vi "S4GUI.vi"(7 "Tab ObsEng":enum32{"Obs", "CCD modes", "Eng"}(tab)) -> ()   [LabVIEW 2018] (continued)
            n1389 = call-dynamic "Read InfoCCDmode.vi"("error in (no error)"=w2404, "S4GUI in"=w2402) -> ("error out"=w2386:errorcluster, "InfoCCDmode"=w2403:T2, "S4GUI out"=w2387:refnum<class "S4GUI.lvclass">)  [unwired: 7 in]
            n1390 = local write "InfoCCDmode"(w2403) -> ()
            n1391 = call-dynamic "CalcTemp.vi"("error in (no error)"=w2386, "S4GUI in"=w2387) -> ("error out"=w2385:errorcluster, "S4GUI out"=w2383:refnum<class "S4GUI.lvclass">)  [unwired: 8 in]
            n1392 = call-dynamic "Read Prev Temp.vi"("error in (no error)"=w2385, "S4GUI in"=w2383) -> ("error out"=w2384:errorcluster, "Prev Temp"=w2381:dbl, "S4GUI out"=w2382:refnum<class "S4GUI.lvclass">)  [unwired: 7 in]
            n1393 = local write "Preview Temp."(w2381) -> ()
          }
          frame "Eng" {
            w2530 = T12."Disabled and Grayed Out" ("Disabled")
            # "Desabilita os botões SET."
            # "Entrou na aba  \"Eng\", ajusta para modo usuário normal..."
            n1394 = local write "password"("" ("password")) -> ()
            n1395 = call-dynamic "Write mode Adm.vi"("error in (no error)"=w2532, "mode Adm"=FALSE, "S4GUI in"=w2533) -> ("error out"=w2525:errorcluster, "S4GUI out"=w2528:refnum<class "S4GUI.lvclass">)  [unwired: 7 in]
            n1396 = property on="Set from Input ch1" class="Bool"("DisabledEnum"=w2530) -> ()  [unwired: 2 in, 2 out]
            n1397 = property on="Set from Input ch3" class="Bool"("DisabledEnum"=w2530) -> ()  [unwired: 2 in, 2 out]
            n1398 = property on="Set from Input ch2" class="Bool"("DisabledEnum"=w2530) -> ()  [unwired: 2 in, 2 out]
            n1399 = property on="Set from Input ch4" class="Bool"("DisabledEnum"=w2530) -> ()  [unwired: 2 in, 2 out]
            n1400 = local read "TARGET NAME WPSEL"() -> (w2481:enum16{"NONE", "OFF", "L/2", "L/4"})
            n1401 = call "Read Instrument.lvclass.vi"("error in (no error)"=w2525, "S4ACS_GUI in"=w2528) -> ("error out"=w2506:errorcluster, "Instrument.lvclass"=w2523:refnum<class "Instrument.lvclass">, "S4ACS_GUI out"=w2527:refnum<class "S4GUI.lvclass">)  [unwired: 7 in]
            n1402 = local read "TARGET NAME CALW"() -> (w2471:T9)
            n1403 = property on="TARGET NAME WPSEL" class="Enum (strict)"() -> ("RingText.Text"=w2479:string)  [unwired: 2 in, 2 out]
            n1404 = call "Read WPSEL.vi"("error in (no error)"=w2506, "Instrument in"=w2523) -> ("error out"=w2521:errorcluster, "Opt_Selector.lvclass"=w2519:refnum<class "Opt_Selector.lvclass">, "Instrument out"=w2522:refnum<class "Instrument.lvclass">)  [unwired: 7 in]
            n1405 = Build Array(-1.0 ("element"), 80.0 ("element"), 0.0 ("element"), 160.0 ("element")) -> (w2482:dbl[])
            n1406 = property on="TARGET NAME CALW" class="Enum (strict)"() -> ("RingText.Text"=w2470:string)  [unwired: 2 in, 2 out]
            n1407 = Build Array(-1.0 ("element"), 0.0 ("element"), 72.0 ("element"), 144.0 ("element"), 216.0 ("element"), 288.0 ("element")) -> (w2474:dbl[])
            n1408 = Index Array "Index Array"(array=w2482, index=w2481) -> (element=w2480:dbl)
            n1409 = call "Write target name.vi"("error in (no error)"=w2521, "target name"=w2479, "Optics in"=w2519) -> ("error out"=w2520:errorcluster, "Optics out"=w2518:refnum<class "Opt_Selector.lvclass">)  [unwired: 7 in]
            n1410 = Index Array(array=w2474, index=w2471) -> (element=w2469:dbl)
            n1411 = call "Write target.vi"("error in (no error)"=w2520, "target"=w2480, "Optics in"=w2518) -> ("error out"=w2516:errorcluster, "Optics out"=w2517:refnum<class "Opt_Selector.lvclass">)  [unwired: 7 in]
            n1412 = call "Write WPSEL.vi"("error in (no error)"=w2516, "Opt_Selector.lvclass"=w2517, "Instrument in"=w2522) -> ("error out"=w2515:errorcluster, "Instrument out"=w2514:refnum<class "Instrument.lvclass">)  [unwired: 7 in]
            n1413 = call "Read CALW.vi"("error in (no error)"=w2515, "Instrument in"=w2514) -> ("error out"=w2512:errorcluster, "Opt_Selector.lvclass"=w2510:refnum<class "Opt_Selector.lvclass">, "Instrument out"=w2507:refnum<class "Instrument.lvclass">)  [unwired: 7 in]
            n1414 = call "Write target name.vi"("error in (no error)"=w2512, "target name"=w2470, "Optics in"=w2510) -> ("error out"=w2513:errorcluster, "Optics out"=w2509:refnum<class "Opt_Selector.lvclass">)  [unwired: 7 in]
            n1415 = call "Write target.vi"("error in (no error)"=w2513, "target"=w2469, "Optics in"=w2509) -> ("error out"=w2511:errorcluster, "Optics out"=w2508:refnum<class "Opt_Selector.lvclass">)  [unwired: 7 in]
            n1416 = local read "TARGET NAME ASEL"() -> (w2463:enum16{"NONE", "OFF", "ON"})
            n1417 = call "Write CALW.vi"("error in (no error)"=w2511, "Opt_Selector.lvclass"=w2508, "Instrument in"=w2507) -> ("error out"=w2503:errorcluster, "Instrument out"=w2504:refnum<class "Instrument.lvclass">)  [unwired: 7 in]
            n1418 = property on="TARGET NAME ASEL" class="Enum (strict)"() -> ("RingText.Text"=w2464:string)  [unwired: 2 in, 2 out]
            n1419 = Build Array(-1.0 ("element"), 0.0 ("element"), 30.0 ("element")) -> (w2465:dbl[])
            n1420 = Index Array(array=w2465, index=w2463) -> (element=w2462:dbl)
            n1421 = call "Read ASEL.vi"("error in (no error)"=w2503, "Instrument in"=w2504) -> ("error out"=w2502:errorcluster, "Opt_Selector.lvclass"=w2500:refnum<class "Opt_Selector.lvclass">, "Instrument out"=w2497:refnum<class "Instrument.lvclass">)  [unwired: 7 in]
            n1422 = call "Write target name.vi"("error in (no error)"=w2502, "target name"=w2464, "Optics in"=w2500) -> ("error out"=w2505:errorcluster, "Optics out"=w2499:refnum<class "Opt_Selector.lvclass">)  [unwired: 7 in]
            n1423 = call "Write target.vi"("error in (no error)"=w2505, "target"=w2462, "Optics in"=w2499) -> ("error out"=w2501:errorcluster, "Optics out"=w2498:refnum<class "Opt_Selector.lvclass">)  [unwired: 7 in]
            n1424 = call "Write ASEL.vi"("error in (no error)"=w2501, "Opt_Selector.lvclass"=w2498, "Instrument in"=w2497) -> ("error out"=w2496:errorcluster, "Instrument out"=w2495:refnum<class "Instrument.lvclass">)  [unwired: 7 in]
            n1425 = local read "GMIR_target"() -> (w2456:dbl)
            n1426 = local read "GFOC_target"() -> (w2457:dbl)
            n1427 = call "Read GFOC.vi"("error in (no error)"=w2496, "Instrument in"=w2495) -> ("error out"=w2460:errorcluster, "Opt_Continuous.lvclass"=w2461:refnum<class "Opt_Continuous.lvclass">, "Instrument out"=w2492:refnum<class "Instrument.lvclass">)  [unwired: 7 in]
            n1428 = call "Write target.vi"("error in (no error)"=w2460, "target"=w2457, "Optics in"=w2461) -> ("error out"=w2494:errorcluster, "Optics out"=w2491:refnum<class "Opt_Continuous.lvclass">)  [unwired: 7 in]
            n1429 = call "Write GFOC.vi"("error in (no error)"=w2494, "Opt_Continuous.lvclass"=w2491, "Instrument in"=w2492) -> ("error out"=w2493:errorcluster, "Instrument out"=w2490:refnum<class "Instrument.lvclass">)  [unwired: 7 in]
            n1430 = call "Read GMIR.vi"("error in (no error)"=w2493, "Instrument in"=w2490) -> ("error out"=w2458:errorcluster, "Opt_Continuous.lvclass"=w2459:refnum<class "Opt_Continuous.lvclass">, "Instrument out"=w2489:refnum<class "Instrument.lvclass">)  [unwired: 7 in]
            n1431 = call "Write target.vi"("error in (no error)"=w2458, "target"=w2456, "Optics in"=w2459) -> ("error out"=w2487:errorcluster, "Optics out"=w2488:refnum<class "Opt_Continuous.lvclass">)  [unwired: 7 in]
            n1432 = local read "TARGET NAME WPROT"() -> (w2425:T10)
            n1433 = call "Write GMIR.vi"("error in (no error)"=w2487, "Opt_Continuous.lvclass"=w2488, "Instrument in"=w2489) -> ("error out"=w2452:errorcluster, "Instrument out"=w2451:refnum<class "Instrument.lvclass">)  [unwired: 7 in]
            n1434 = property on="TARGET NAME WPROT" class="Enum (strict)"() -> ("RingText.Text"=w2424:string)  [unwired: 2 in, 2 out]
            n1435 = call "Read WPROT.vi"("error in (no error)"=w2452, "Instrument in"=w2451) -> ("error out"=w2449:errorcluster, "Opt_Selector.lvclass"=w2453:refnum<class "Opt_Selector.lvclass">, "Instrument out"=w2450:refnum<class "Instrument.lvclass">)  [unwired: 7 in]
            n1436 = Build Array(-1.0 ("element"), 0.0 ("element"), 22.5 ("element"), 45.0 ("element"), 67.5 ("element"), 90.0 ("element"), 112.5 ("element"), 135.0 ("element"), 157.5 ("element"), 180.0 ("element"), 202.5 ("element"), 225.0 ("element"), 247.5 ("element"), 270.0 ("element"), 292.5 ("element"), 315.0 ("element"), 337.5 ("element")) -> (w2438:dbl[])
            n1437 = Index Array(array=w2438, index=w2425) -> (element=w2426:dbl)
            n1438 = call "Write target name.vi"("error in (no error)"=w2449, "target name"=w2424, "Optics in"=w2453) -> ("error out"=w2448:errorcluster, "Optics out"=w2455:refnum<class "Opt_Selector.lvclass">)  [unwired: 7 in]
            n1439 = call "Write target.vi"("error in (no error)"=w2448, "target"=w2426, "Optics in"=w2455) -> ("error out"=w2447:errorcluster, "Optics out"=w2454:refnum<class "Opt_Selector.lvclass">)  [unwired: 7 in]
            n1440 = call "Write WPROT.vi"("error in (no error)"=w2447, "Opt_Selector.lvclass"=w2454, "Instrument in"=w2450) -> ("error out"=w2445:errorcluster, "Instrument out"=w2446:refnum<class "Instrument.lvclass">)  [unwired: 7 in]
            n1441 = call "Write Instrument.lvclass.vi"("error in (no error)"=w2445, "Instrument.lvclass"=w2446, "S4ACS_GUI in"=w2527) -> ("error out"=w2524:errorcluster, "S4ACS_GUI out"=w2526:refnum<class "S4GUI.lvclass">)  [unwired: 7 in]
          }
          frame Default {
          }
        }
      }
      event "S4ICS protocol": Value Change {
        # "2024-04-04: Não se usa mais o ID para configurar a comunicação..."
        # "TCP-IP"
        # "ZeroMQ"
        # "Inicializar nova comunicação, de acordo\n com valor de S4ICS mode\n\nServer.Write id (T=13 ou F=5)\nInstrument.Init"
        # "Parar a comunciação atual\nServer.End"
        n1442 = event-data() -> ("NewVal"=w2538:bool)  [unwired: 1 in, 5 out]
        n1443 = call "Read Instrument.lvclass.vi"("error in (no error)"=w2548, "S4ACS_GUI in"=w2549) -> ("error out"=w2543:errorcluster, "Instrument.lvclass"=w2546:refnum<class "Instrument.lvclass">, "S4ACS_GUI out"=w2547:refnum<class "S4GUI.lvclass">)  [unwired: 7 in]
        n1444 = call-dynamic "End.vi"("error in (no error)"=w2543, "Server in"=w2546) -> ("error out"=w2542:errorcluster, "Server out"=w2545:refnum<class "Instrument.lvclass">)  [unwired: 8 in]
        n1445 = Select(t=u32 13, s=w2538, f=u32 5) -> (s? t:f=w2552:u32)
        n1446 = call-dynamic "Write id.vi"("error in (no error)"=w2542, "id"=w2552, "Server in"=w2545) -> ("error out"=w2541:errorcluster, "Server out"=w2544:refnum<class "Instrument.lvclass">)  [unwired: 7 in]
        n1447 = call-dynamic "Initialize.vi"("error in (no error)"=w2541, "Instrument in"=w2544) -> ("error out"=w2539:errorcluster, "Instrument out"=w2540:refnum<class "Instrument.lvclass">)  [unwired: 8 in]
        n1448 = call "Write Instrument.lvclass.vi"("error in (no error)"=w2539, "Instrument.lvclass"=w2540, "S4ACS_GUI in"=w2547) -> ("error out"=w2536:errorcluster, "S4ACS_GUI out"=w2537:refnum<class "S4GUI.lvclass">)  [unwired: 7 in]
      }
      event "Set from Input ch1": Value Change {
        # "ACS"
        # "GUI"
        # "EM_MODE = E.M."
        # "Readou Rate:\n30         0\n20         1     \n10         2\n1           3"
        # "EM_MODE = Conv"
        # "Readou Rate:\n1         0\n0.1      1"
        # "Readou Rate:\n1         0\n0.1      1     \n10       2\n20       3\n30       4"
        n1449 = event-data() -> ()  [unwired: 1 in, 6 out]
        n1450 = local read "Input Cluster"() -> (w2577:T8)
        n1451 = Unbundle By Name(w2577) -> ("Parameters"=w2576:T5)
        n1452 = Unbundle By Name(w2576) -> ("Image \nInitial Line"=w2604:u16, "Image\nInitial Column"=w2603:u16, "Image\nFinal Line"=w2602:u16, "Image\nFInal Column"=w2601:u16, "Vertical\nBinning"=w2600:u16, "Horizontal\nBinning"=w2599:u16, "Pre-amplification\nGain"=w2598:u8, "CCD\nEM Gain"=w2597:u16, "Readout\nRate"=w2596:u8, "Shutter\nOpenning Time"=w2595:i32, "Shutter\nClosing Time"=w2594:i32, "Vertical\nShift Speed"=w2593:u8, "Read\nMode"=w2592:u8, "Vertical\nClock Voltage"=w2591:u8, "A/D \nChannel"=w2590:u32, "Shutter\nMode"=w2589:u16, "Shutter\nTTL"=w2588:u16, "Trigger\nMode"=w2587:u16, "Frame\nTransfer"=w2568:bool, "Acquisition\nMode"=w2586:u8, "CCD \nEM Mode"=w2585:u8)
        n1453 = call-dynamic "Write User Event.vi"("error in (no error)"=w2556, "User Event"="SET CCD CONFIG CHANNEL1 ", "S4GUI in"=w2557) -> ("error out"=w2554:errorcluster, "S4GUI out"=w2555:refnum<class "S4GUI.lvclass">)  [unwired: 7 in]
        n1454 = call-dynamic "Read AcquisitionA.vi"("error in (no error)"=w2554, "S4ACS_GUI in"=w2555) -> ("error out"=w2620:errorcluster, "Acquisition.lvclass"=w2623:refnum<class "Acquisition.lvclass">, "S4ACS_GUI out"=w2624:refnum<class "S4GUI.lvclass">)  [unwired: 7 in]
        n1455 = call-dynamic "Read Channel.vi"("error in (no error)"=w2620, "Acquisition in"=w2623) -> ("error out"=w2619:errorcluster, "Channel.lvclass"=w2621:refnum<class "Channel.lvclass">, "Acquisition out"=w2622:refnum<class "Acquisition.lvclass">)  [unwired: 7 in]
        n1456 = call-dynamic "Read Interface.vi"("error in (no error)"=w2619, "Channel in"=w2621) -> ("error out"=w2567:errorcluster, "Interface.lvclass"=w2569:refnum<class "Interface.lvclass">, "Channel out"=w2564:refnum<class "Channel.lvclass">)  [unwired: 7 in]
        n1457 = call-dynamic "Write PREV_FT.vi"("error in (no error)"=w2567, "PREV_FT"=w2568, "Interface in"=w2569) -> ("error out"=w2566:errorcluster, "Interface out"=w2565:refnum<class "Interface.lvclass">)  [unwired: 7 in]
        n1458 = call-dynamic "Read target cluster.vi"("error in (no error)"=w2566, "Channel in"=w2564) -> ("error out"=w2562:errorcluster, "target cluster"=w2560:T30, "Channel out"=w2561:refnum<class "Channel.lvclass">)  [unwired: 7 in]
        n1459 = Bundle By Name(cluster=w2560, "INITIAL_LINE"=w2604, "INITIAL_COLUMN"=w2603, "FINAL_LINE"=w2602, "FINAL_COLUMN"=w2601, "VBIN"=w2600, "HBIN"=w2599, "PREAMP"=w2598, "EM_GAIN"=w2597, "READOUT_RATE"=w2596, "SHUTTER_OPENING_TIME"=w2595, "SHUTTER_CLOSING_TIME"=w2594, "VERTICAL_SHIFT_SPEED"=w2593, "READ_MODE"=w2592, "VERTICAL_CLOCK_VOLTAGE"=w2591, "AD_CHANNEL"=w2590, "SHUTTER_MODE"=w2589, "SHUTTER_TTL"=w2588, "TRIGGER_MODE"=w2587, "FRAME_TRANSFER"=w2568, "ACQUISITION_MODE"=w2586, "EM_MODE"=w2585) -> (w2559:T30)
        n1460 = call-dynamic "Write target cluster.vi"("error in (no error)"=w2562, "target cluster"=w2559, "Channel in"=w2561) -> ("error out"=w2558:errorcluster, "Channel out"=w2563:refnum<class "Channel.lvclass">)  [unwired: 7 in]
        n1461 = Flatten To String(anything=w2559, error in (no error)=w2558) -> (data string=w2608:string, error out=w2607:errorcluster)  [unwired: 2 in, 1 out]
        n1462 = call "Write flatted cluster.vi"("error in (no error)"=w2607, "flatted cluster"=w2608, "Interface in"=w2565) -> ("error out"=w2606:errorcluster, "Interface out"=w2605:refnum<class "Interface.lvclass">)  [unwired: 7 in]
        n1463 = call-dynamic "Write Interface.vi"("error in (no error)"=w2606, "Interface.lvclass"=w2605, "Channel in"=w2563) -> ("error out"=w2580:errorcluster, "Channel out"=w2583:refnum<class "Channel.lvclass">)  [unwired: 7 in]
        n1464 = call "Write section_name.vi"("error in (no error)"=w2580, "section_name"="CCD_ACS1", "Channel in"=w2583) -> ("error out"=w2579:errorcluster, "Channel out"=w2582:refnum<class "Channel.lvclass">)  [unwired: 7 in]
        n1465 = call-dynamic "save config.vi"("error in (no error)"=w2579, "file config"="lastsaved.cfg", "Channel in"=w2582) -> ("error out"=w2578:errorcluster, "Channel out"=w2581:refnum<class "Channel.lvclass">)  [unwired: 7 in]
        n1466 = call-dynamic "Read State Machine.vi"("error in (no error)"=w2578, "Device in"=w2581) -> ("error out"=w2615:errorcluster, "State Machine.lvclass"=w2617:refnum<class "State Machine.lvclass">, "Device out"=w2618:refnum<class "Channel.lvclass">)  [unwired: 7 in]
        n1467 = call-dynamic "Write State.vi"("error in (no error)"=w2615, "State"=60, "State Machine in"=w2617) -> ("error out"=w2614:errorcluster, "State Machine out"=w2616:refnum<class "State Machine.lvclass">)  [unwired: 7 in]
        n1468 = call-dynamic "Write State Machine.vi"("error in (no error)"=w2614, "State Machine.lvclass"=w2616, "Device in"=w2618) -> ("error out"=w2611:errorcluster, "Device out"=w2612:refnum<class "Channel.lvclass">)  [unwired: 7 in]
        n1469 = call-dynamic "Write Channel.vi"("error in (no error)"=w2611, "Channel.lvclass"=w2612, "Acquisition in"=w2622) -> ("error out"=w2610:errorcluster, "Acquisition out"=w2609:refnum<class "Acquisition.lvclass">)  [unwired: 7 in]
        n1470 = call-dynamic "Write AcquisitionA.vi"("error in (no error)"=w2610, "Acquisition.lvclass"=w2609, "S4ACS_GUI in"=w2624) -> ("error out"=w2571:errorcluster, "S4ACS_GUI out"=w2572:refnum<class "S4GUI.lvclass">)  [unwired: 7 in]
        n1471 = call "Write cfg file.vi"("error in (no error)"=w2571, "cfg file"="lastsaved.cfg", "S4ACS_GUI in"=w2572) -> ("error out"=w2574:errorcluster, "S4ACS_GUI out"=w2575:refnum<class "S4GUI.lvclass">)  [unwired: 7 in]
      }
      event "Input Cluster.Parameters.CCD \nEM Mode": Value Change {
        n1472 = event-data() -> ()  [unwired: 1 in, 6 out]
        n1473 = local read "Input Cluster"() -> (w2639:T8)
        n1474 = Unbundle By Name(w2639) -> ("Parameters"=w2640:T5)
        n1475 = Unbundle By Name(w2640) -> ("Readout\nRate"=→"Readout\nRate":u8, "CCD \nEM Mode"=w2634:u8)
        n1476 = case shown="0, Default" w2634 {
          tunnel: [string[] ["30 MHz", "20 MHz", "10 MHz", "1 MHz"] ("Strings []") string[] ["1 MHz", "0.1 MHz"] ("Strings []")] -> w2633
          tunnel: [u8 3 u8 0] -> w2632
          frame 0, Default {
          }
          frame 1 {
          }
        }
        n1477 = local read "Cameras Cluster"() -> (w2627:T7)
        n1478 = flat-sequence {
          tunnel: w2632 -> [w2642]
          tunnel: w2633 -> [w2641]
          tunnel: w2634 -> [w2643]
          tunnel: [w2643] -> w2631
          tunnel: [w2642] -> w2629
          tunnel: w2640 -> [w2649]
          tunnel: [w2648] -> w2638
          tunnel: w2631 -> [w2644]
          tunnel: w2629 -> [w2645]
          tunnel: w2628 -> [w2647]
          tunnel: [w2646] -> w2626
          frame #0 {
            n1479 = property on="Readout\nRate" class="Ring (strict)"("Strings []"=w2641) -> ()  [unwired: 2 in, 2 out]
            n1480 = property on="Readout Rate" class="Ring (strict)"("Strings []"=w2641) -> ()  [unwired: 2 in, 2 out]
            n1481 = property on="Readout Rate 4" class="Ring (strict)"("Strings []"=w2641) -> ()  [unwired: 2 in, 2 out]
            n1482 = property on="Readout Rate 2" class="Ring (strict)"("Strings []"=w2641) -> ()  [unwired: 2 in, 2 out]
            n1483 = property on="Readout Rate 3" class="Ring (strict)"("Strings []"=w2641) -> ()  [unwired: 2 in, 2 out]
          }
          frame #1 {
            n1484 = Bundle By Name(cluster=w2647, "Readout Rate"=w2645, "Read Mode"=w2644) -> (w2646:T31)
            n1485 = Bundle By Name(cluster=w2649, "Readout\nRate"=w2645, "CCD \nEM Mode"=w2644) -> (w2648:T5)
          }
        }
        n1486 = Unbundle By Name(w2627) -> ("Current Configuration"=w2628:T31)
        n1487 = Bundle By Name(cluster=w2639, "Parameters"=w2638) -> (w2637:T8)
        n1488 = local write "Input Cluster"(w2637) -> ()
        n1489 = Bundle By Name(cluster=w2627, "Current Configuration"=w2626) -> (w2625:T7)
        n1490 = local write "Cameras Cluster"(w2625) -> ()
      }
      event "Set from Input ch2": Value Change {
        n1491 = event-data() -> ()  [unwired: 1 in, 6 out]
        n1492 = local read "Input Cluster"() -> (w2678:T8)
        n1493 = Unbundle By Name(w2678) -> ("Parameters"=w2677:T5)
        n1494 = call-dynamic "Write User Event.vi"("error in (no error)"=w2656, "User Event"="SET CCD CONFIG CHANNEL2 ", "S4GUI in"=w2657) -> ("error out"=w2654:errorcluster, "S4GUI out"=w2655:refnum<class "S4GUI.lvclass">)  [unwired: 7 in]
        n1495 = Unbundle By Name(w2677) -> ("Image \nInitial Line"=w2705:u16, "Image\nInitial Column"=w2704:u16, "Image\nFinal Line"=w2703:u16, "Image\nFInal Column"=w2702:u16, "Vertical\nBinning"=w2701:u16, "Horizontal\nBinning"=w2700:u16, "Pre-amplification\nGain"=w2699:u8, "CCD\nEM Gain"=w2698:u16, "Readout\nRate"=w2697:u8, "Shutter\nOpenning Time"=w2696:i32, "Shutter\nClosing Time"=w2695:i32, "Vertical\nShift Speed"=w2694:u8, "Read\nMode"=w2693:u8, "Vertical\nClock Voltage"=w2692:u8, "A/D \nChannel"=w2691:u32, "Shutter\nMode"=w2690:u16, "Shutter\nTTL"=w2689:u16, "Trigger\nMode"=w2688:u16, "Frame\nTransfer"=w2668:bool, "Acquisition\nMode"=w2687:u8, "CCD \nEM Mode"=w2686:u8)
        n1496 = call "Read AcquisitionB.vi"("error in (no error)"=w2654, "S4ACS_GUI in"=w2655) -> ("error out"=w2721:errorcluster, "Acquisition.lvclass"=w2724:refnum<class "Acquisition.lvclass">, "S4ACS_GUI out"=w2725:refnum<class "S4GUI.lvclass">)  [unwired: 7 in]
        n1497 = call-dynamic "Read Channel.vi"("error in (no error)"=w2721, "Acquisition in"=w2724) -> ("error out"=w2720:errorcluster, "Channel.lvclass"=w2722:refnum<class "Channel.lvclass">, "Acquisition out"=w2723:refnum<class "Acquisition.lvclass">)  [unwired: 7 in]
        n1498 = call-dynamic "Read Interface.vi"("error in (no error)"=w2720, "Channel in"=w2722) -> ("error out"=w2669:errorcluster, "Interface.lvclass"=w2670:refnum<class "Interface.lvclass">, "Channel out"=w2665:refnum<class "Channel.lvclass">)  [unwired: 7 in]
        n1499 = call-dynamic "Write PREV_FT.vi"("error in (no error)"=w2669, "PREV_FT"=w2668, "Interface in"=w2670) -> ("error out"=w2662:errorcluster, "Interface out"=w2660:refnum<class "Interface.lvclass">)  [unwired: 7 in]
        n1500 = call-dynamic "Read target cluster.vi"("error in (no error)"=w2662, "Channel in"=w2665) -> ("error out"=w2667:errorcluster, "target cluster"=w2664:T30, "Channel out"=w2666:refnum<class "Channel.lvclass">)  [unwired: 7 in]
        n1501 = Bundle By Name(cluster=w2664, "INITIAL_LINE"=w2705, "INITIAL_COLUMN"=w2704, "FINAL_LINE"=w2703, "FINAL_COLUMN"=w2702, "VBIN"=w2701, "HBIN"=w2700, "PREAMP"=w2699, "EM_GAIN"=w2698, "READOUT_RATE"=w2697, "SHUTTER_OPENING_TIME"=w2696, "SHUTTER_CLOSING_TIME"=w2695, "VERTICAL_SHIFT_SPEED"=w2694, "READ_MODE"=w2693, "VERTICAL_CLOCK_VOLTAGE"=w2692, "AD_CHANNEL"=w2691, "SHUTTER_MODE"=w2690, "SHUTTER_TTL"=w2689, "TRIGGER_MODE"=w2688, "FRAME_TRANSFER"=w2668, "ACQUISITION_MODE"=w2687, "EM_MODE"=w2686) -> (w2663:T30)
        n1502 = call-dynamic "Write target cluster.vi"("error in (no error)"=w2667, "target cluster"=w2663, "Channel in"=w2666) -> ("error out"=w2661:errorcluster, "Channel out"=w2659:refnum<class "Channel.lvclass">)  [unwired: 7 in]
        n1503 = Flatten To String(anything=w2663, error in (no error)=w2661) -> (data string=w2709:string, error out=w2708:errorcluster)  [unwired: 2 in, 1 out]
        n1504 = call "Write flatted cluster.vi"("error in (no error)"=w2708, "flatted cluster"=w2709, "Interface in"=w2660) -> ("error out"=w2707:errorcluster, "Interface out"=w2706:refnum<class "Interface.lvclass">)  [unwired: 7 in]
        n1505 = call-dynamic "Write Interface.vi"("error in (no error)"=w2707, "Interface.lvclass"=w2706, "Channel in"=w2659) -> ("error out"=w2681:errorcluster, "Channel out"=w2684:refnum<class "Channel.lvclass">)  [unwired: 7 in]
        n1506 = call "Write section_name.vi"("error in (no error)"=w2681, "section_name"="CCD_ACS2", "Channel in"=w2684) -> ("error out"=w2680:errorcluster, "Channel out"=w2683:refnum<class "Channel.lvclass">)  [unwired: 7 in]
        n1507 = call-dynamic "save config.vi"("error in (no error)"=w2680, "file config"="lastsaved.cfg", "Channel in"=w2683) -> ("error out"=w2679:errorcluster, "Channel out"=w2682:refnum<class "Channel.lvclass">)  [unwired: 7 in]
        n1508 = call-dynamic "Read State Machine.vi"("error in (no error)"=w2679, "Device in"=w2682) -> ("error out"=w2716:errorcluster, "State Machine.lvclass"=w2718:refnum<class "State Machine.lvclass">, "Device out"=w2719:refnum<class "Channel.lvclass">)  [unwired: 7 in]
        n1509 = call-dynamic "Write State.vi"("error in (no error)"=w2716, "State"=60, "State Machine in"=w2718) -> ("error out"=w2715:errorcluster, "State Machine out"=w2717:refnum<class "State Machine.lvclass">)  [unwired: 7 in]
        n1510 = call-dynamic "Write State Machine.vi"("error in (no error)"=w2715, "State Machine.lvclass"=w2717, "Device in"=w2719) -> ("error out"=w2712:errorcluster, "Device out"=w2713:refnum<class "Channel.lvclass">)  [unwired: 7 in]
        n1511 = call-dynamic "Write Channel.vi"("error in (no error)"=w2712, "Channel.lvclass"=w2713, "Acquisition in"=w2723) -> ("error out"=w2711:errorcluster, "Acquisition out"=w2710:refnum<class "Acquisition.lvclass">)  [unwired: 7 in]
        n1512 = call "Write AcquisitionB.vi"("error in (no error)"=w2711, "Acquisition.lvclass"=w2710, "S4ACS_GUI in"=w2725) -> ("error out"=w2671:errorcluster, "S4ACS_GUI out"=w2672:refnum<class "S4GUI.lvclass">)  [unwired: 7 in]
        n1513 = call "Write cfg file.vi"("error in (no error)"=w2671, "cfg file"="lastsaved.cfg", "S4ACS_GUI in"=w2672) -> ("error out"=w2674:errorcluster, "S4ACS_GUI out"=w2675:refnum<class "S4GUI.lvclass">)  [unwired: 7 in]
      }
      event "Set from Input ch3": Value Change {
        n1514 = event-data() -> ()  [unwired: 1 in, 6 out]
        n1515 = local read "Input Cluster"() -> (w2750:T8)
        n1516 = Unbundle By Name(w2750) -> ("Parameters"=w2749:T5)
        n1517 = call-dynamic "Write User Event.vi"("error in (no error)"=w2728, "User Event"="SET CCD CONFIG CHANNEL 3 ", "S4GUI in"=w2729) -> ("error out"=w2726:errorcluster, "S4GUI out"=w2727:refnum<class "S4GUI.lvclass">)  [unwired: 7 in]
        n1518 = Unbundle By Name(w2749) -> ("Image \nInitial Line"=w2777:u16, "Image\nInitial Column"=w2776:u16, "Image\nFinal Line"=w2775:u16, "Image\nFInal Column"=w2774:u16, "Vertical\nBinning"=w2773:u16, "Horizontal\nBinning"=w2772:u16, "Pre-amplification\nGain"=w2771:u8, "CCD\nEM Gain"=w2770:u16, "Readout\nRate"=w2769:u8, "Shutter\nOpenning Time"=w2768:i32, "Shutter\nClosing Time"=w2767:i32, "Vertical\nShift Speed"=w2766:u8, "Read\nMode"=w2765:u8, "Vertical\nClock Voltage"=w2764:u8, "A/D \nChannel"=w2763:u32, "Shutter\nMode"=w2762:u16, "Shutter\nTTL"=w2761:u16, "Trigger\nMode"=w2760:u16, "Frame\nTransfer"=w2740:bool, "Acquisition\nMode"=w2759:u8, "CCD \nEM Mode"=w2758:u8)
        n1519 = call-dynamic "Read AcquisitionC.vi"("error in (no error)"=w2726, "S4ACS_GUI in"=w2727) -> ("error out"=w2793:errorcluster, "Acquisition.lvclass"=w2796:refnum<class "Acquisition.lvclass">, "S4ACS_GUI out"=w2797:refnum<class "S4GUI.lvclass">)  [unwired: 7 in]
        n1520 = call-dynamic "Read Channel.vi"("error in (no error)"=w2793, "Acquisition in"=w2796) -> ("error out"=w2792:errorcluster, "Channel.lvclass"=w2794:refnum<class "Channel.lvclass">, "Acquisition out"=w2795:refnum<class "Acquisition.lvclass">)  [unwired: 7 in]
        n1521 = call-dynamic "Read Interface.vi"("error in (no error)"=w2792, "Channel in"=w2794) -> ("error out"=w2741:errorcluster, "Interface.lvclass"=w2742:refnum<class "Interface.lvclass">, "Channel out"=w2737:refnum<class "Channel.lvclass">)  [unwired: 7 in]
        n1522 = call-dynamic "Write PREV_FT.vi"("error in (no error)"=w2741, "PREV_FT"=w2740, "Interface in"=w2742) -> ("error out"=w2731:errorcluster, "Interface out"=w2738:refnum<class "Interface.lvclass">)  [unwired: 7 in]
        n1523 = call-dynamic "Read target cluster.vi"("error in (no error)"=w2731, "Channel in"=w2737) -> ("error out"=w2739:errorcluster, "target cluster"=w2733:T30, "Channel out"=w2736:refnum<class "Channel.lvclass">)  [unwired: 7 in]
        n1524 = Bundle By Name(cluster=w2733, "INITIAL_LINE"=w2777, "INITIAL_COLUMN"=w2776, "FINAL_LINE"=w2775, "FINAL_COLUMN"=w2774, "VBIN"=w2773, "HBIN"=w2772, "PREAMP"=w2771, "EM_GAIN"=w2770, "READOUT_RATE"=w2769, "SHUTTER_OPENING_TIME"=w2768, "SHUTTER_CLOSING_TIME"=w2767, "VERTICAL_SHIFT_SPEED"=w2766, "READ_MODE"=w2765, "VERTICAL_CLOCK_VOLTAGE"=w2764, "AD_CHANNEL"=w2763, "SHUTTER_MODE"=w2762, "SHUTTER_TTL"=w2761, "TRIGGER_MODE"=w2760, "FRAME_TRANSFER"=w2740, "ACQUISITION_MODE"=w2759, "EM_MODE"=w2758) -> (w2732:T30)
        n1525 = call-dynamic "Write target cluster.vi"("error in (no error)"=w2739, "target cluster"=w2732, "Channel in"=w2736) -> ("error out"=w2734:errorcluster, "Channel out"=w2735:refnum<class "Channel.lvclass">)  [unwired: 7 in]
        n1526 = Flatten To String(anything=w2732, error in (no error)=w2734) -> (data string=w2781:string, error out=w2780:errorcluster)  [unwired: 2 in, 1 out]
        n1527 = call "Write flatted cluster.vi"("error in (no error)"=w2780, "flatted cluster"=w2781, "Interface in"=w2738) -> ("error out"=w2779:errorcluster, "Interface out"=w2778:refnum<class "Interface.lvclass">)  [unwired: 7 in]
        n1528 = call-dynamic "Write Interface.vi"("error in (no error)"=w2779, "Interface.lvclass"=w2778, "Channel in"=w2735) -> ("error out"=w2753:errorcluster, "Channel out"=w2756:refnum<class "Channel.lvclass">)  [unwired: 7 in]
        n1529 = call "Write section_name.vi"("error in (no error)"=w2753, "section_name"="CCD_ACS3", "Channel in"=w2756) -> ("error out"=w2752:errorcluster, "Channel out"=w2755:refnum<class "Channel.lvclass">)  [unwired: 7 in]
        n1530 = call-dynamic "save config.vi"("error in (no error)"=w2752, "file config"="lastsaved.cfg", "Channel in"=w2755) -> ("error out"=w2751:errorcluster, "Channel out"=w2754:refnum<class "Channel.lvclass">)  [unwired: 7 in]
        n1531 = call-dynamic "Read State Machine.vi"("error in (no error)"=w2751, "Device in"=w2754) -> ("error out"=w2788:errorcluster, "State Machine.lvclass"=w2790:refnum<class "State Machine.lvclass">, "Device out"=w2791:refnum<class "Channel.lvclass">)  [unwired: 7 in]
        n1532 = call-dynamic "Write State.vi"("error in (no error)"=w2788, "State"=60, "State Machine in"=w2790) -> ("error out"=w2787:errorcluster, "State Machine out"=w2789:refnum<class "State Machine.lvclass">)  [unwired: 7 in]
        n1533 = call-dynamic "Write State Machine.vi"("error in (no error)"=w2787, "State Machine.lvclass"=w2789, "Device in"=w2791) -> ("error out"=w2784:errorcluster, "Device out"=w2785:refnum<class "Channel.lvclass">)  [unwired: 7 in]
        n1534 = call-dynamic "Write Channel.vi"("error in (no error)"=w2784, "Channel.lvclass"=w2785, "Acquisition in"=w2795) -> ("error out"=w2783:errorcluster, "Acquisition out"=w2782:refnum<class "Acquisition.lvclass">)  [unwired: 7 in]
        n1535 = call-dynamic "Write AcquisitionC.vi"("error in (no error)"=w2783, "Acquisition.lvclass"=w2782, "S4ACS_GUI in"=w2797) -> ("error out"=w2743:errorcluster, "S4ACS_GUI out"=w2744:refnum<class "S4GUI.lvclass">)  [unwired: 7 in]
        n1536 = call "Write cfg file.vi"("error in (no error)"=w2743, "cfg file"="lastsaved.cfg", "S4ACS_GUI in"=w2744) -> ("error out"=w2746:errorcluster, "S4ACS_GUI out"=w2747:refnum<class "S4GUI.lvclass">)  [unwired: 7 in]
      }
      event "Set from Input ch4": Value Change {
        n1537 = event-data() -> ()  [unwired: 1 in, 6 out]
        n1538 = local read "Input Cluster"() -> (w2822:T8)
        n1539 = Unbundle By Name(w2822) -> ("Parameters"=w2821:T5)
        n1540 = call-dynamic "Write User Event.vi"("error in (no error)"=w2801, "User Event"="SET CCD CONFIG CHANNEL4 ", "S4GUI in"=w2800) -> ("error out"=w2798:errorcluster, "S4GUI out"=w2799:refnum<class "S4GUI.lvclass">)  [unwired: 7 in]
        n1541 = Unbundle By Name(w2821) -> ("Image \nInitial Line"=w2849:u16, "Image\nInitial Column"=w2848:u16, "Image\nFinal Line"=w2847:u16, "Image\nFInal Column"=w2846:u16, "Vertical\nBinning"=w2845:u16, "Horizontal\nBinning"=w2844:u16, "Pre-amplification\nGain"=w2843:u8, "CCD\nEM Gain"=w2842:u16, "Readout\nRate"=w2841:u8, "Shutter\nOpenning Time"=w2840:i32, "Shutter\nClosing Time"=w2839:i32, "Vertical\nShift Speed"=w2838:u8, "Read\nMode"=w2837:u8, "Vertical\nClock Voltage"=w2836:u8, "A/D \nChannel"=w2835:u32, "Shutter\nMode"=w2834:u16, "Shutter\nTTL"=w2833:u16, "Trigger\nMode"=w2832:u16, "Frame\nTransfer"=w2812:bool, "Acquisition\nMode"=w2831:u8, "CCD \nEM Mode"=w2830:u8)
        n1542 = call-dynamic "Read AcquisitionD.vi"("error in (no error)"=w2798, "S4ACS_GUI in"=w2799) -> ("error out"=w2865:errorcluster, "Acquisition.lvclass"=w2868:refnum<class "Acquisition.lvclass">, "S4ACS_GUI out"=w2869:refnum<class "S4GUI.lvclass">)  [unwired: 7 in]
        n1543 = call-dynamic "Read Channel.vi"("error in (no error)"=w2865, "Acquisition in"=w2868) -> ("error out"=w2864:errorcluster, "Channel.lvclass"=w2866:refnum<class "Channel.lvclass">, "Acquisition out"=w2867:refnum<class "Acquisition.lvclass">)  [unwired: 7 in]
        n1544 = call-dynamic "Read Interface.vi"("error in (no error)"=w2864, "Channel in"=w2866) -> ("error out"=w2813:errorcluster, "Interface.lvclass"=w2814:refnum<class "Interface.lvclass">, "Channel out"=w2809:refnum<class "Channel.lvclass">)  [unwired: 7 in]
        n1545 = call-dynamic "Write PREV_FT.vi"("error in (no error)"=w2813, "PREV_FT"=w2812, "Interface in"=w2814) -> ("error out"=w2804:errorcluster, "Interface out"=w2810:refnum<class "Interface.lvclass">)  [unwired: 7 in]
        n1546 = call-dynamic "Read target cluster.vi"("error in (no error)"=w2804, "Channel in"=w2809) -> ("error out"=w2811:errorcluster, "target cluster"=w2808:T30, "Channel out"=w2807:refnum<class "Channel.lvclass">)  [unwired: 7 in]
        n1547 = Bundle By Name(cluster=w2808, "INITIAL_LINE"=w2849, "INITIAL_COLUMN"=w2848, "FINAL_LINE"=w2847, "FINAL_COLUMN"=w2846, "VBIN"=w2845, "HBIN"=w2844, "PREAMP"=w2843, "EM_GAIN"=w2842, "READOUT_RATE"=w2841, "SHUTTER_OPENING_TIME"=w2840, "SHUTTER_CLOSING_TIME"=w2839, "VERTICAL_SHIFT_SPEED"=w2838, "READ_MODE"=w2837, "VERTICAL_CLOCK_VOLTAGE"=w2836, "AD_CHANNEL"=w2835, "SHUTTER_MODE"=w2834, "SHUTTER_TTL"=w2833, "TRIGGER_MODE"=w2832, "FRAME_TRANSFER"=w2812, "ACQUISITION_MODE"=w2831, "EM_MODE"=w2830) -> (w2806:T30)
        n1548 = call-dynamic "Write target cluster.vi"("error in (no error)"=w2811, "target cluster"=w2806, "Channel in"=w2807) -> ("error out"=w2805:errorcluster, "Channel out"=w2803:refnum<class "Channel.lvclass">)  [unwired: 7 in]
        n1549 = Flatten To String(anything=w2806, error in (no error)=w2805) -> (data string=w2853:string, error out=w2852:errorcluster)  [unwired: 2 in, 1 out]
        n1550 = call "Write flatted cluster.vi"("error in (no error)"=w2852, "flatted cluster"=w2853, "Interface in"=w2810) -> ("error out"=w2851:errorcluster, "Interface out"=w2850:refnum<class "Interface.lvclass">)  [unwired: 7 in]
        n1551 = call-dynamic "Write Interface.vi"("error in (no error)"=w2851, "Interface.lvclass"=w2850, "Channel in"=w2803) -> ("error out"=w2825:errorcluster, "Channel out"=w2828:refnum<class "Channel.lvclass">)  [unwired: 7 in]
        n1552 = call "Write section_name.vi"("error in (no error)"=w2825, "section_name"="CCD_ACS4", "Channel in"=w2828) -> ("error out"=w2824:errorcluster, "Channel out"=w2827:refnum<class "Channel.lvclass">)  [unwired: 7 in]
        n1553 = call-dynamic "save config.vi"("error in (no error)"=w2824, "file config"="lastsaved.cfg", "Channel in"=w2827) -> ("error out"=w2823:errorcluster, "Channel out"=w2826:refnum<class "Channel.lvclass">)  [unwired: 7 in]
        n1554 = call-dynamic "Read State Machine.vi"("error in (no error)"=w2823, "Device in"=w2826) -> ("error out"=w2860:errorcluster, "State Machine.lvclass"=w2862:refnum<class "State Machine.lvclass">, "Device out"=w2863:refnum<class "Channel.lvclass">)  [unwired: 7 in]
        n1555 = call-dynamic "Write State.vi"("error in (no error)"=w2860, "State"=60, "State Machine in"=w2862) -> ("error out"=w2859:errorcluster, "State Machine out"=w2861:refnum<class "State Machine.lvclass">)  [unwired: 7 in]
        n1556 = call-dynamic "Write State Machine.vi"("error in (no error)"=w2859, "State Machine.lvclass"=w2861, "Device in"=w2863) -> ("error out"=w2856:errorcluster, "Device out"=w2857:refnum<class "Channel.lvclass">)  [unwired: 7 in]
        n1557 = call-dynamic "Write Channel.vi"("error in (no error)"=w2856, "Channel.lvclass"=w2857, "Acquisition in"=w2867) -> ("error out"=w2855:errorcluster, "Acquisition out"=w2854:refnum<class "Acquisition.lvclass">)  [unwired: 7 in]
        n1558 = call-dynamic "Write AcquisitionD.vi"("error in (no error)"=w2855, "Acquisition.lvclass"=w2854, "S4ACS_GUI in"=w2869) -> ("error out"=w2815:errorcluster, "S4ACS_GUI out"=w2816:refnum<class "S4GUI.lvclass">)  [unwired: 7 in]
        n1559 = call "Write cfg file.vi"("error in (no error)"=w2815, "cfg file"="lastsaved.cfg", "S4ACS_GUI in"=w2816) -> ("error out"=w2818:errorcluster, "S4ACS_GUI out"=w2819:refnum<class "S4GUI.lvclass">)  [unwired: 7 in]
      }
      event "Restore Default ch1": Value Change {
        n1560 = event-data() -> ()  [unwired: 1 in, 6 out]
        n1561 = call-dynamic "Read AcquisitionA.vi"("error in (no error)"=w2900, "S4ACS_GUI in"=w2901) -> ("error out"=w2896:errorcluster, "Acquisition.lvclass"=w2898:refnum<class "Acquisition.lvclass">, "S4ACS_GUI out"=w2899:refnum<class "S4GUI.lvclass">)  [unwired: 7 in]
        n1562 = call-dynamic "Read Channel.vi"("error in (no error)"=w2896, "Acquisition in"=w2898) -> ("error out"=w2883:errorcluster, "Channel.lvclass"=w2885:refnum<class "Channel.lvclass">, "Acquisition out"=w2897:refnum<class "Acquisition.lvclass">)  [unwired: 7 in]
        n1563 = call "Write section_name.vi"("error in (no error)"=w2883, "section_name"="CCD_ACS1", "Channel in"=w2885) -> ("error out"=w2882:errorcluster, "Channel out"=w2884:refnum<class "Channel.lvclass">)  [unwired: 7 in]
        n1564 = call-dynamic "load config.vi"("error in (no error)"=w2882, "cfg file name"="default.cfg", "Channel in"=w2884) -> ("error out"=w2880:errorcluster, "Channel out"=w2881:refnum<class "Channel.lvclass">)  [unwired: 7 in]
        n1565 = call-dynamic "Read State Machine.vi"("error in (no error)"=w2880, "Device in"=w2881) -> ("error out"=w2892:errorcluster, "State Machine.lvclass"=w2894:refnum<class "State Machine.lvclass">, "Device out"=w2895:refnum<class "Channel.lvclass">)  [unwired: 7 in]
        n1566 = call-dynamic "Write State.vi"("error in (no error)"=w2892, "State"=60, "State Machine in"=w2894) -> ("error out"=w2891:errorcluster, "State Machine out"=w2893:refnum<class "State Machine.lvclass">)  [unwired: 7 in]
        n1567 = call-dynamic "Write State Machine.vi"("error in (no error)"=w2891, "State Machine.lvclass"=w2893, "Device in"=w2895) -> ("error out"=w2876:errorcluster, "Device out"=w2872:refnum<class "Channel.lvclass">)  [unwired: 7 in]
        n1568 = call "Write section_name.vi"("error in (no error)"=w2876, "section_name"="CCD_ACS1", "Channel in"=w2872) -> ("error out"=w2877:errorcluster, "Channel out"=w2871:refnum<class "Channel.lvclass">)  [unwired: 7 in]
        n1569 = call-dynamic "save config.vi"("error in (no error)"=w2877, "file config"="lastsaved.cfg", "Channel in"=w2871) -> ("error out"=w2875:errorcluster, "Channel out"=w2870:refnum<class "Channel.lvclass">)  [unwired: 7 in]
        n1570 = call-dynamic "Write Channel.vi"("error in (no error)"=w2875, "Channel.lvclass"=w2870, "Acquisition in"=w2897) -> ("error out"=w2889:errorcluster, "Acquisition out"=w2888:refnum<class "Acquisition.lvclass">)  [unwired: 7 in]
        n1571 = call-dynamic "Write AcquisitionA.vi"("error in (no error)"=w2889, "Acquisition.lvclass"=w2888, "S4ACS_GUI in"=w2899) -> ("error out"=w2887:errorcluster, "S4ACS_GUI out"=w2878:refnum<class "S4GUI.lvclass">)  [unwired: 7 in]
      }
      event "Load Button": Value Change {
        n1572 = event-data() -> ()  [unwired: 1 in, 6 out]
        n1573 = call <vilib>:"Application Directory.vi"() -> ("Application Directory"=w2913:path)
        n1574 = call "File Dialog"("start path"=w2913, "prompt"="Select file...", "button label"="Open", "default name"="lastsaved.cfg", "error in"=w2907, "pattern (all files)"="*.cfg") -> ("selected path"=w2905:path, "cancelled"=w2908:bool, "error out"=→"error out 2":errorcluster)  [unwired: 6 in, 1 out]
        "selected path" <- w2905
        n1575 = Path To String(path=w2905) -> (string=w2904:string)
        n1576 = Match Pattern(string=w2904, regular expression="SPARC4_GUI\\") -> (after substring=w2902:string)  [unwired: 1 in, 3 out]
        n1577 = case shown="False" w2908 {
          tunnel: w2916 -> [w3025 w3027]
          tunnel: [w2941 w3027] -> w2915
          tunnel: [w2939 w3026] -> w2914
          tunnel: w2907 -> [w2938 w3026]
          tunnel: w2902 -> [w2937 _]
          frame False {
            n1578 = call-dynamic "Read AcquisitionA.vi"("error in (no error)"=w2938, "S4ACS_GUI in"=w3025) -> ("error out"=w3021:errorcluster, "Acquisition.lvclass"=w3023:refnum<class "Acquisition.lvclass">, "S4ACS_GUI out"=w3024:refnum<class "S4GUI.lvclass">)  [unwired: 7 in]
            n1579 = call-dynamic "Read Channel.vi"("error in (no error)"=w3021, "Acquisition in"=w3023) -> ("error out"=w3008:errorcluster, "Channel.lvclass"=w3010:refnum<class "Channel.lvclass">, "Acquisition out"=w3022:refnum<class "Acquisition.lvclass">)  [unwired: 7 in]
            n1580 = call "Write section_name.vi"("error in (no error)"=w3008, "section_name"="CCD_ACS1", "Channel in"=w3010) -> ("error out"=w3007:errorcluster, "Channel out"=w3009:refnum<class "Channel.lvclass">)  [unwired: 7 in]
            n1581 = call-dynamic "load config.vi"("error in (no error)"=w3007, "cfg file name"=w2937, "Channel in"=w3009) -> ("error out"=w2933:errorcluster, "Channel out"=w2935:refnum<class "Channel.lvclass">)  [unwired: 7 in]
            n1582 = call-dynamic "save config.vi"("error in (no error)"=w2933, "file config"="lastsaved.cfg", "Channel in"=w2935) -> ("error out"=w2936:errorcluster, "Channel out"=w2934:refnum<class "Channel.lvclass">)  [unwired: 7 in]
            n1583 = call-dynamic "Read State Machine.vi"("error in (no error)"=w2936, "Device in"=w2934) -> ("error out"=w3017:errorcluster, "State Machine.lvclass"=w3019:refnum<class "State Machine.lvclass">, "Device out"=w3020:refnum<class "Channel.lvclass">)  [unwired: 7 in]
            n1584 = call-dynamic "Write State.vi"("error in (no error)"=w3017, "State"=60, "State Machine in"=w3019) -> ("error out"=w3016:errorcluster, "State Machine out"=w3018:refnum<class "State Machine.lvclass">)  [unwired: 7 in]
            n1585 = call-dynamic "Write State Machine.vi"("error in (no error)"=w3016, "State Machine.lvclass"=w3018, "Device in"=w3020) -> ("error out"=w3013:errorcluster, "Device out"=w3014:refnum<class "Channel.lvclass">)  [unwired: 7 in]
            n1586 = call-dynamic "Write Channel.vi"("error in (no error)"=w3013, "Channel.lvclass"=w3014, "Acquisition in"=w3022) -> ("error out"=w3012:errorcluster, "Acquisition out"=w3011:refnum<class "Acquisition.lvclass">)  [unwired: 7 in]
            n1587 = call-dynamic "Write AcquisitionA.vi"("error in (no error)"=w3012, "Acquisition.lvclass"=w3011, "S4ACS_GUI in"=w3024) -> ("error out"=w2948:errorcluster, "S4ACS_GUI out"=w2947:refnum<class "S4GUI.lvclass">)  [unwired: 7 in]
            n1588 = call "Read AcquisitionB.vi"("error in (no error)"=w2948, "S4ACS_GUI in"=w2947) -> ("error out"=w2990:errorcluster, "Acquisition.lvclass"=w2988:refnum<class "Acquisition.lvclass">, "S4ACS_GUI out"=w2987:refnum<class "S4GUI.lvclass">)  [unwired: 7 in]
            n1589 = call-dynamic "Read Channel.vi"("error in (no error)"=w2990, "Acquisition in"=w2988) -> ("error out"=w3003:errorcluster, "Channel.lvclass"=w3001:refnum<class "Channel.lvclass">, "Acquisition out"=w2989:refnum<class "Acquisition.lvclass">)  [unwired: 7 in]
            n1590 = call "Write section_name.vi"("error in (no error)"=w3003, "section_name"="CCD_ACS2", "Channel in"=w3001) -> ("error out"=w3004:errorcluster, "Channel out"=w3002:refnum<class "Channel.lvclass">)  [unwired: 7 in]
            n1591 = call-dynamic "load config.vi"("error in (no error)"=w3004, "cfg file name"=w2937, "Channel in"=w3002) -> ("error out"=w2930:errorcluster, "Channel out"=w2928:refnum<class "Channel.lvclass">)  [unwired: 7 in]
            n1592 = call-dynamic "save config.vi"("error in (no error)"=w2930, "file config"="lastsaved.cfg", "Channel in"=w2928) -> ("error out"=w2929:errorcluster, "Channel out"=w2927:refnum<class "Channel.lvclass">)  [unwired: 7 in]
            n1593 = call-dynamic "Read State Machine.vi"("error in (no error)"=w2929, "Device in"=w2927) -> ("error out"=w2994:errorcluster, "State Machine.lvclass"=w2992:refnum<class "State Machine.lvclass">, "Device out"=w2991:refnum<class "Channel.lvclass">)  [unwired: 7 in]
            n1594 = call-dynamic "Write State.vi"("error in (no error)"=w2994, "State"=60, "State Machine in"=w2992) -> ("error out"=w2995:errorcluster, "State Machine out"=w2993:refnum<class "State Machine.lvclass">)  [unwired: 7 in]
            n1595 = call-dynamic "Write State Machine.vi"("error in (no error)"=w2995, "State Machine.lvclass"=w2993, "Device in"=w2991) -> ("error out"=w2998:errorcluster, "Device out"=w2997:refnum<class "Channel.lvclass">)  [unwired: 7 in]
            n1596 = call-dynamic "Write Channel.vi"("error in (no error)"=w2998, "Channel.lvclass"=w2997, "Acquisition in"=w2989) -> ("error out"=w2999:errorcluster, "Acquisition out"=w3000:refnum<class "Acquisition.lvclass">)  [unwired: 7 in]
            n1597 = call "Write AcquisitionB.vi"("error in (no error)"=w2999, "Acquisition.lvclass"=w3000, "S4ACS_GUI in"=w2987) -> ("error out"=w2946:errorcluster, "S4ACS_GUI out"=w2945:refnum<class "S4GUI.lvclass">)  [unwired: 7 in]
            n1598 = call-dynamic "Read AcquisitionC.vi"("error in (no error)"=w2946, "S4ACS_GUI in"=w2945) -> ("error out"=w2983:errorcluster, "Acquisition.lvclass"=w2985:refnum<class "Acquisition.lvclass">, "S4ACS_GUI out"=w2986:refnum<class "S4GUI.lvclass">)  [unwired: 7 in]
            n1599 = call-dynamic "Read Channel.vi"("error in (no error)"=w2983, "Acquisition in"=w2985) -> ("error out"=w2970:errorcluster, "Channel.lvclass"=w2972:refnum<class "Channel.lvclass">, "Acquisition out"=w2984:refnum<class "Acquisition.lvclass">)  [unwired: 7 in]
            n1600 = call "Write section_name.vi"("error in (no error)"=w2970, "section_name"="CCD_ACS3", "Channel in"=w2972) -> ("error out"=w2969:errorcluster, "Channel out"=w2971:refnum<class "Channel.lvclass">)  [unwired: 7 in]
            n1601 = call-dynamic "load config.vi"("error in (no error)"=w2969, "cfg file name"=w2937, "Channel in"=w2971) -> ("error out"=w2925:errorcluster, "Channel out"=w2923:refnum<class "Channel.lvclass">)  [unwired: 7 in]
            n1602 = call-dynamic "save config.vi"("error in (no error)"=w2925, "file config"="lastsaved.cfg", "Channel in"=w2923) -> ("error out"=w2924:errorcluster, "Channel out"=w2922:refnum<class "Channel.lvclass">)  [unwired: 7 in]
            n1603 = call-dynamic "Read State Machine.vi"("error in (no error)"=w2924, "Device in"=w2922) -> ("error out"=w2979:errorcluster, "State Machine.lvclass"=w2981:refnum<class "State Machine.lvclass">, "Device out"=w2982:refnum<class "Channel.lvclass">)  [unwired: 7 in]
            n1604 = call-dynamic "Write State.vi"("error in (no error)"=w2979, "State"=60, "State Machine in"=w2981) -> ("error out"=w2978:errorcluster, "State Machine out"=w2980:refnum<class "State Machine.lvclass">)  [unwired: 7 in]
            n1605 = call-dynamic "Write State Machine.vi"("error in (no error)"=w2978, "State Machine.lvclass"=w2980, "Device in"=w2982) -> ("error out"=w2975:errorcluster, "Device out"=w2976:refnum<class "Channel.lvclass">)  [unwired: 7 in]
            n1606 = call-dynamic "Write Channel.vi"("error in (no error)"=w2975, "Channel.lvclass"=w2976, "Acquisition in"=w2984) -> ("error out"=w2974:errorcluster, "Acquisition out"=w2973:refnum<class "Acquisition.lvclass">)  [unwired: 7 in]
            n1607 = call-dynamic "Write AcquisitionC.vi"("error in (no error)"=w2974, "Acquisition.lvclass"=w2973, "S4ACS_GUI in"=w2986) -> ("error out"=w2944:errorcluster, "S4ACS_GUI out"=w2943:refnum<class "S4GUI.lvclass">)  [unwired: 7 in]
            n1608 = call-dynamic "Read AcquisitionD.vi"("error in (no error)"=w2944, "S4ACS_GUI in"=w2943) -> ("error out"=w2952:errorcluster, "Acquisition.lvclass"=w2950:refnum<class "Acquisition.lvclass">, "S4ACS_GUI out"=w2949:refnum<class "S4GUI.lvclass">)  [unwired: 7 in]
            n1609 = call-dynamic "Read Channel.vi"("error in (no error)"=w2952, "Acquisition in"=w2950) -> ("error out"=w2965:errorcluster, "Channel.lvclass"=w2963:refnum<class "Channel.lvclass">, "Acquisition out"=w2951:refnum<class "Acquisition.lvclass">)  [unwired: 7 in]
            n1610 = call "Write section_name.vi"("error in (no error)"=w2965, "section_name"="CCD_ACS4", "Channel in"=w2963) -> ("error out"=w2966:errorcluster, "Channel out"=w2964:refnum<class "Channel.lvclass">)  [unwired: 7 in]
            n1611 = call-dynamic "load config.vi"("error in (no error)"=w2966, "cfg file name"=w2937, "Channel in"=w2964) -> ("error out"=w2921:errorcluster, "Channel out"=w2919:refnum<class "Channel.lvclass">)  [unwired: 7 in]
            n1612 = call-dynamic "save config.vi"("error in (no error)"=w2921, "file config"="lastsaved.cfg", "Channel in"=w2919) -> ("error out"=w2920:errorcluster, "Channel out"=w2918:refnum<class "Channel.lvclass">)  [unwired: 7 in]
            n1613 = call-dynamic "Read State Machine.vi"("error in (no error)"=w2920, "Device in"=w2918) -> ("error out"=w2956:errorcluster, "State Machine.lvclass"=w2954:refnum<class "State Machine.lvclass">, "Device out"=w2953:refnum<class "Channel.lvclass">)  [unwired: 7 in]
            n1614 = call-dynamic "Write State.vi"("error in (no error)"=w2956, "State"=60, "State Machine in"=w2954) -> ("error out"=w2957:errorcluster, "State Machine out"=w2955:refnum<class "State Machine.lvclass">)  [unwired: 7 in]
            n1615 = call-dynamic "Write State Machine.vi"("error in (no error)"=w2957, "State Machine.lvclass"=w2955, "Device in"=w2953) -> ("error out"=w2960:errorcluster, "Device out"=w2959:refnum<class "Channel.lvclass">)  [unwired: 7 in]
            n1616 = call-dynamic "Write Channel.vi"("error in (no error)"=w2960, "Channel.lvclass"=w2959, "Acquisition in"=w2951) -> ("error out"=w2961:errorcluster, "Acquisition out"=w2962:refnum<class "Acquisition.lvclass">)  [unwired: 7 in]
            n1617 = call-dynamic "Write AcquisitionD.vi"("error in (no error)"=w2961, "Acquisition.lvclass"=w2962, "S4ACS_GUI in"=w2949) -> ("error out"=w2940:errorcluster, "S4ACS_GUI out"=w2942:refnum<class "S4GUI.lvclass">)  [unwired: 7 in]
            n1618 = call "Write cfg file.vi"("error in (no error)"=w2940, "cfg file"=w2937, "S4ACS_GUI in"=w2942) -> ("error out"=w2939:errorcluster, "S4ACS_GUI out"=w2941:refnum<class "S4GUI.lvclass">)  [unwired: 7 in]
          }
          frame True {
          }
        }
      }
      event "Save As Button": Value Change {
        n1619 = event-data() -> ()  [unwired: 1 in, 6 out]
        n1620 = call <vilib>:"Application Directory.vi"() -> ("Application Directory"=w3039:path)
        n1621 = call "File Dialog2"("start path"=w3039, "prompt"="Select file...", "button label"="Save", "default name"="lastsaved.cfg", "error in"=w3033, "pattern (all files)"="*.cfg") -> ("selected path"=w3031:path, "cancelled"=w3034:bool, "error out"=→"error out 3":errorcluster)  [unwired: 6 in, 1 out]
        n1622 = Path To String(path=w3031) -> (string=w3030:string)
        n1623 = Match Pattern(string=w3030, regular expression="SPARC4_GUI\\") -> (after substring=w3028:string)  [unwired: 1 in, 3 out]
        n1624 = case shown="False" w3034 {
          tunnel: w3042 -> [w3107 w3109]
          tunnel: [w3055 w3109] -> w3041
          tunnel: [w3053 w3108] -> w3040
          tunnel: w3033 -> [w3052 w3108]
          tunnel: w3028 -> [w3051 _]
          frame False {
            n1625 = call-dynamic "Read AcquisitionA.vi"("error in (no error)"=w3052, "S4ACS_GUI in"=w3107) -> ("error out"=w3103:errorcluster, "Acquisition.lvclass"=w3105:refnum<class "Acquisition.lvclass">, "S4ACS_GUI out"=w3106:refnum<class "S4GUI.lvclass">)  [unwired: 7 in]
